vi "getDeviceClockChannel.vi"(8 "error in (no error)":errorcluster, 10 "device":refnum<class "device.lvclass">, 11 "deviceDataBase in":refnum<class "deviceDataBase.lvclass">) -> (0 "error out":errorcluster, 1 "isClock":bool, 2 "timingChannel":refnum<class "Channel.lvclass">, 3 "deviceDataBase out":refnum<class "deviceDataBase.lvclass">, 4 "noChannel":bool)   [LabVIEW 2011, in "Tools.lvlib" / "DatabaseHelpers.lvlib" / "deviceDataBase.lvclass"]
uses:
  deviceDataBase.lvclass
  Database Objects/device/device.lvclass
  Database Objects/Channel/Channel.lvclass
  Database Objects/ChannelArray/ChannelArray.lvclass
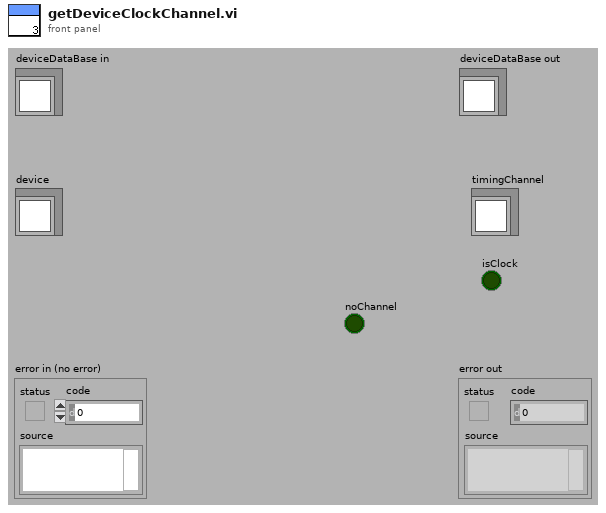
[diagram p1: front panel]
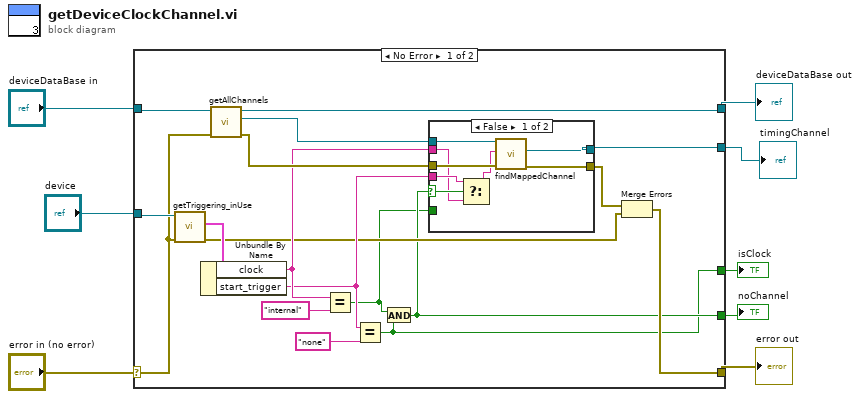
[diagram p0: block diagram]
diagram:
  n1 = case shown="No Error" "error in (no error)" {
    selector: "error in (no error)" -> [w21 w37]
    tunnel: [w18 w37] -> w7
    tunnel: [w20 w36] -> w5
    tunnel: "deviceDataBase in" -> [w24 w36]
    tunnel: "device" -> [w26 _]
    tunnel: [w19 _] -> w3
    tunnel: [w11 _] -> w2
    tunnel: [w9 _] -> w1
    frame No Error {
      n2 = call "getTriggering_inUse.vi"("error in (no error)"=w21, "device.lvclass in"=w26) -> ("error out"=w12:errorcluster, "triggering_inUse"=w25:cluster{"start_trigger":string, "clock":string})  [unwired: 7 in, 1 out]
      n3 = Unbundle By Name(w25) -> ("clock"=w16:string, "start_trigger"=w14:string)
      n4 = call "getAllChannels.vi"("error in (no error)"=w21, "deviceDataBase in"=w24) -> ("error out"=w22:errorcluster, "ChannelArray.lvclass"=w23:refnum<class "ChannelArray.lvclass">, "deviceDataBase out"=w20:refnum<class "deviceDataBase.lvclass">)  [unwired: 7 in]
      n5 = Equal?(x=w16, y="internal") -> (x = y?=w10:bool)
      n6 = Equal?(x=w14, y="none") -> (x = y?=w9:bool)
      n7 = And(x=w10, y=w9) -> (x .and. y?=w11:bool)
      n8 = case shown="False" w11 {
        selector: w11 -> [w30 _]
        tunnel: w23 -> [w34 _]
        tunnel: w22 -> [w33 w35]
        tunnel: [w32 _] -> w19
        tunnel: w16 -> [w27 _]
        tunnel: w10 -> [_ _]
        tunnel: w14 -> [w28 _]
        tunnel: [w31 w35] -> w13
        frame False {
          n9 = Select(t=w28, s=w30, f=w27) -> (s? t:f=w29:string)
          n10 = call "findMappedChannel.vi"("error in (no error)"=w33, "name of mappedTo channel"=w29, "ChannelArray in"=w34) -> ("error out"=w31:errorcluster, "Channel"=w32:refnum<class "Channel.lvclass">)  [unwired: 6 in, 1 out]
        }
        frame True {
        }
      }
      n11 = Merge Errors(w13, w12) -> (w18:errorcluster)
    }
    frame Error {
    }
  }
  "error out" <- w7
  "deviceDataBase out" <- w5
  "timingChannel" <- w3
  "noChannel" <- w2
  "isClock" <- w1
